vi "UTIL_MergeData.vi"(9 "Status Code":i32, 10 "New Data":dbl[](array[numeric]), 11 "Data In":dbl[][](array[numeric])) -> (3 "Data out":dbl[][](array[numeric]))   [LabVIEW 2024]
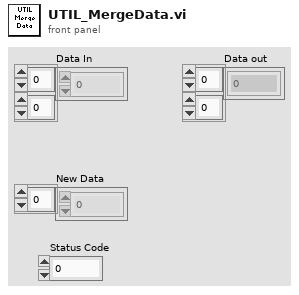
[diagram p1: front panel]
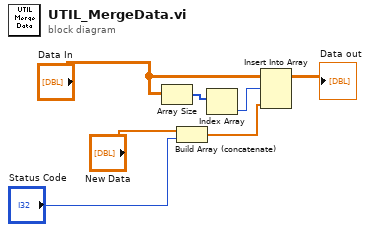
[diagram p0: block diagram]
diagram:
  n1 = Array Size(array="Data In") -> (size(s)=w4:i32[])
  n2 = Build Array (concatenate)("New Data", "Status Code") -> (w6:dbl[])
  n3 = Index Array(array=w4) -> (element=w5:i32)  [unwired: 1 in]
  n4 = Insert Into Array(array="Data In", index (row)=w5, new element=w6) -> (→"Data out":dbl[][])  [unwired: 1 in]
